vi "SinglePoint.vi"(8 "Error In 2":errorcluster, 11 "Async State Vars 2":T1) -> (0 "Error Out":errorcluster, 3 "Async State Vars out":T1)   [LabVIEW 2015, in "Waveform-Processing-Custom-Device Shared.lvlib" / "SinglePoint.lvlib"]
uses:
  SinglePoint.lvlib
  Built/Waveform-Processing-Custom-Device/c/Waveform-Processing-Custom-Device Engine Pharlap.llb/Circular Buffer Operations.ctl
  Built/Waveform-Processing-Custom-Device/c/Waveform-Processing-Custom-Device Engine Pharlap.llb/Circular Buffer.lvlib
  Built/Waveform-Processing-Custom-Device/c/Waveform-Processing-Custom-Device Engine Pharlap.llb/Circular Buffer(2D DBL).vi
  Engine/Types/Async FIFOs.ctl
  Engine/Waveform-Processing-Custom-Device Engine.lvlib
  <vilib>/NI Veristand/Custom Device Waveform API/Single Waveform Read (DBL)/Single Waveform Read (DBL).lvclass
  <vilib>/NI Veristand/Custom Device Waveform API/Single Waveform Write (DBL)/Single Waveform Write (DBL).lvclass
  <vilib>/NI Veristand/Custom Device API/Waveform Data Reference.ctl
  <vilib>/NI VeriStand/Custom Device API/Custom Device API.lvlib
  Engine/Types/Async State Vars.ctl
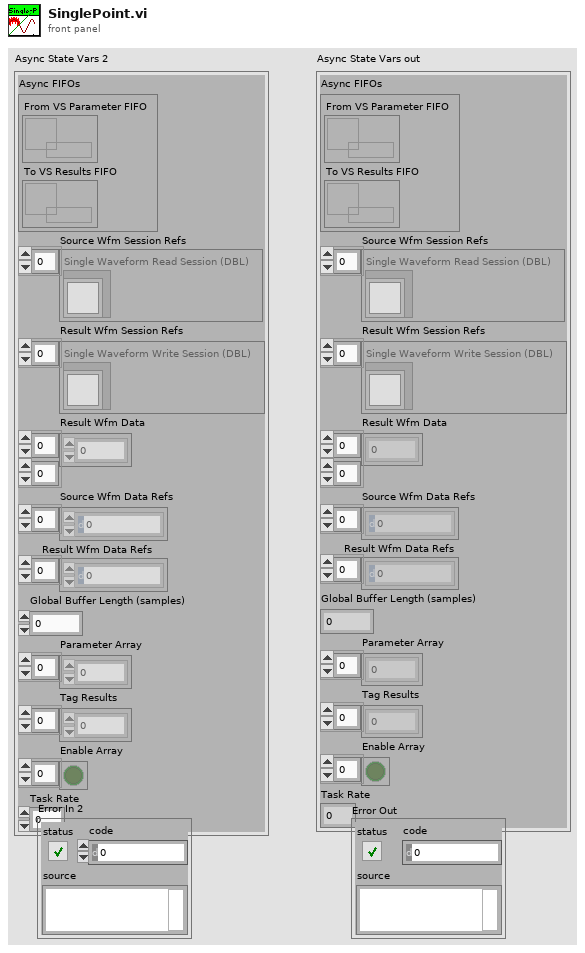
[diagram p1: front panel]
types:
  T1 = typedef "Waveform-Processing-Custom-Device Engine.lvlib/Async State Vars.ctl" = cluster{"Async FIFOs":T2, "Source Wfm Session Refs":refnum<class "Single Waveform Read (DBL).lvclass">[], "Result Wfm Session Refs":refnum<class "Single Waveform Write (DBL).lvclass">[], "Result Wfm Data":dbl[][], "Source Wfm Data Refs":T3[], "Result Wfm Data Refs":T3[], "Global Buffer Length (samples)":dbl, "Parameter Array":dbl[], "Tag Results":dbl[], "Enable Array":bool[], "Task Rate":dbl}
  T2 = typedef "Waveform-Processing-Custom-Device Engine.lvlib/Async FIFOs.ctl" = cluster{"From VS Parameter FIFO":refnum<k33>, "To VS Results FIFO":refnum<k33>}
  T3 = typedef "Custom Device API.lvlib/Waveform Data Reference.ctl" = i32
  T4 = typedef "Circular Buffer.lvlib/Circular Buffer Operations.ctl" = enum16{"Initialize", "Get Backlog", "Write", "Read (continuous)", "Read (most recent)"}
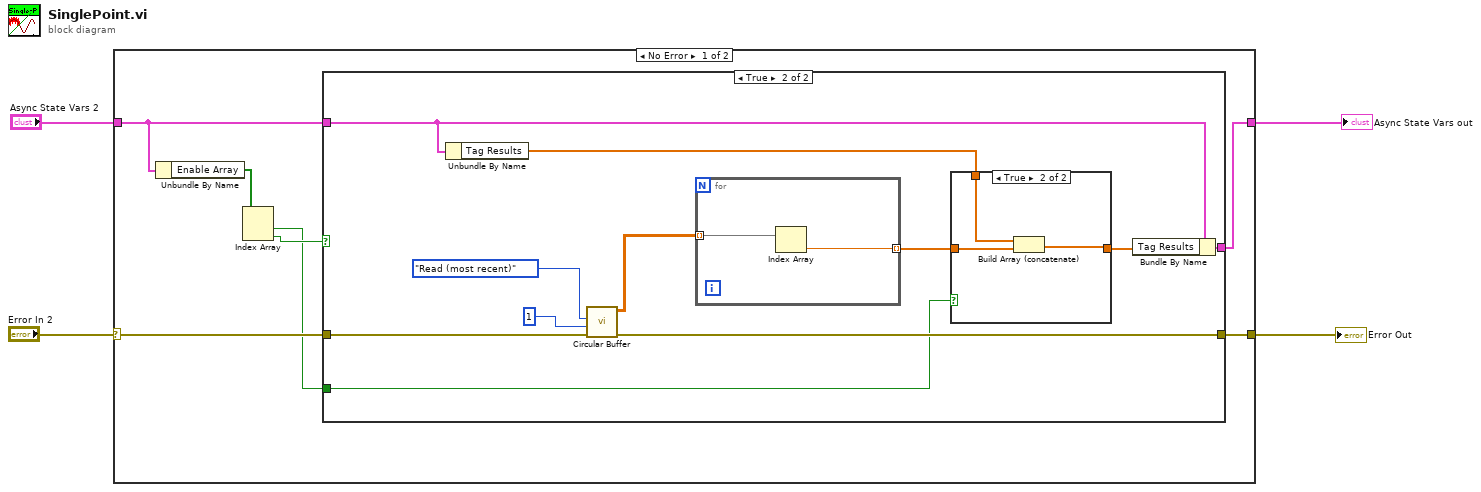
[diagram p0: block diagram]
diagram:
  n1 = case shown="No Error" "Error In 2" {
    selector: "Error In 2" -> [w11 w32]
    tunnel: [w10 w32] -> w2
    tunnel: "Async State Vars 2" -> [w8 w31]
    tunnel: [w9 w31] -> w4
    frame No Error {
      n2 = Unbundle By Name(w8) -> ("Enable Array"=w7:bool[])
      n3 = Index Array(array=w7) -> (element #1=w5:bool, element #2=w6:bool)  [unwired: 2 in]
      n4 = case shown="True" w6 {
        tunnel: w11 -> [w13 w23]
        tunnel: [w13 w22] -> w10
        tunnel: [w12 w21] -> w9
        tunnel: w8 -> [w12 w15]
        tunnel: w5 -> [_ w14]
        frame False {
        }
        frame True {
          n5 = Unbundle By Name(w15) -> ("Tag Results"=w18:dbl[])
          n6 = call-poly <userlib>:"Circular Buffer.vi"("error in (no error)"=w23, "Read Size"=1, "Operation"=Circular_Buffer_Operations."Read (most recent)") -> ("error out"=w22:errorcluster, "Data Out"=w20:dbl[][])  [unwired: 5 in, 2 out]
          n7 = for {
            tunnel: w20 -> [w30] mode=indexing
            tunnel: [w29] -> w17 mode=indexing
            n8 = Index Array(array=w30) -> (element=w29:dbl)  [unwired: 1 in]
          }
          n9 = case shown="True" w14 {
            tunnel: w18 -> [_ w28]
            tunnel: w17 -> [w25 w27]
            tunnel: [w25 w26] -> w16
            frame False {
            }
            frame True {
              n10 = Build Array (concatenate)(w28, w27) -> (w26:dbl[])
            }
          }
          n11 = Bundle By Name(cluster=w15, "Tag Results"=w16) -> (w21:T1)
        }
      }
    }
    frame Error {
    }
  }
  "Error Out" <- w2
  "Async State Vars out" <- w4
